vi "fxp32_16-to-int_mul4.vi"(4 "FXP32_16 4":fxp<+/-,32,16>, 5 "FXP32_16 3":fxp<+/-,32,16>, 6 "FXP32_16 2":fxp<+/-,32,16>, 7 "FXP32_16 1":fxp<+/-,32,16>) -> (0 "32bit integer 4":i32, 1 "32bit integer 3":i32, 2 "32bit integer 2":i32, 3 "32bit integer 1":i32)   [LabVIEW 2018]
uses:
  <vilib>/rvi/FXPMathLib/FxpInterpret/XNode/nifxpmath_Interpret.xnode
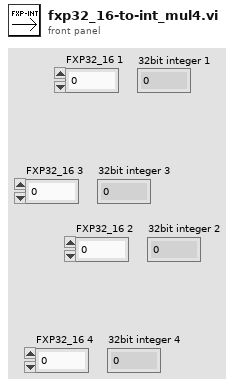
[diagram p1: front panel]
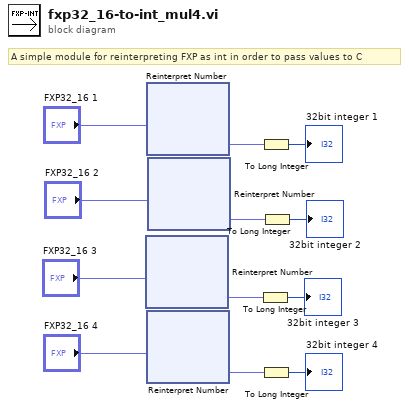
[diagram p0: block diagram]
diagram:
  # "A simple module for reinterpreting FXP as int in order to pass values to C"
  n1 = xnode "Reinterpret Number"("x"="FXP32_16 3") -> ("y"=w5:fxp<+/-,32,32>)
  n2 = xnode "Reinterpret Number"("x"="FXP32_16 1") -> ("y"=w11:fxp<+/-,32,32>)
  n3 = xnode "Reinterpret Number"("x"="FXP32_16 4") -> ("y"=w2:fxp<+/-,32,32>)
  n4 = xnode "Reinterpret Number"("x"="FXP32_16 2") -> ("y"=w8:fxp<+/-,32,32>)
  n5 = To Long Integer(number=w5) -> (32bit integer=→"32bit integer 3":i32)
  n6 = To Long Integer(number=w11) -> (32bit integer=→"32bit integer 1":i32)
  n7 = To Long Integer(number=w2) -> (32bit integer=→"32bit integer 4":i32)
  n8 = To Long Integer(number=w8) -> (32bit integer=→"32bit integer 2":i32)
